vi "Dynamic Channel Lookups.vi"(8 "error in (no error)":errorcluster, 11 "Child Refs":T1[](array[typedef]) format="%.0x") -> (0 "error out":errorcluster, 3 "SLSC Dynamic Inputs":T2[](array[typedef]))   [LabVIEW 2015, in "SLSC-12201 DIO System Explorer.lvlib"]
uses:
  SLSC-12201 DIO System Explorer.lvlib
  Shared/SLSC Dynamic Channel.ctl
  Shared/SLSC Dynamic Channel Type.ctl
  <vilib>/NI Veristand/Custom Device API/Custom Device Item Ref.ctl
  Shared/Constants.vi
  <vilib>/NI Veristand/Custom Device API/Get Item Property (String).vi
  <vilib>/regexp/Match Regular Expression.xnode
  <vilib>/NI Veristand/Custom Device API/Custom Device API.lvlib
  Shared/SLSC-12201 DIO Shared.lvlib
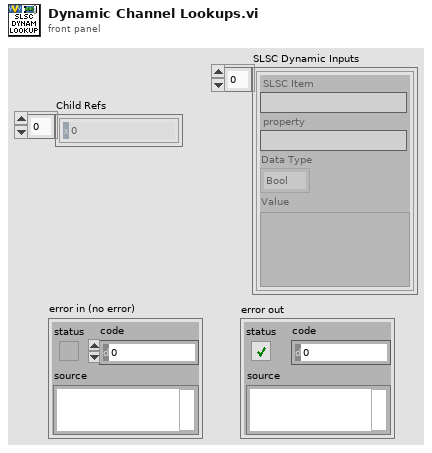
[diagram p1: front panel]
types:
  T1 = typedef "Custom Device API.lvlib/Custom Device Item Ref.ctl" = u64
  T2 = typedef "SLSC-12201 DIO Shared.lvlib/SLSC Dynamic Channel.ctl" = cluster{"SLSC Item":string, "property":string, "Data Type":T3, "Value":variant}
  T3 = typedef "SLSC-12201 DIO Shared.lvlib/SLSC Dynamic Channel Type.ctl" = enum16{"Bool", "Double", "I32", "I64", "String", "U32", "U64", "EnumI32"}
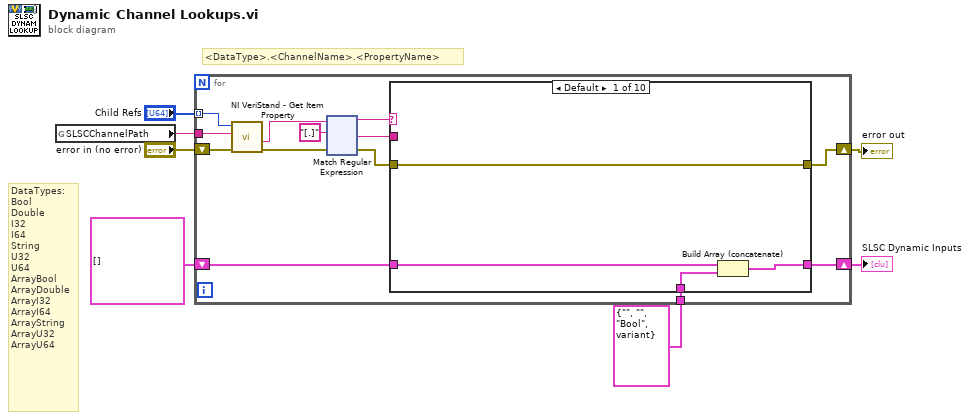
[diagram p0: block diagram]
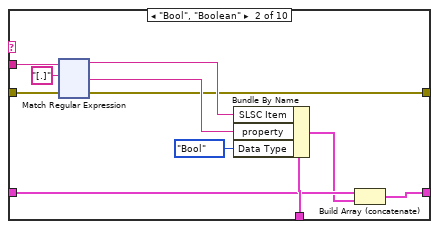
[diagram p2: hidden frame]
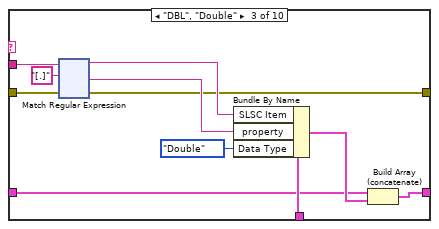
[diagram p3: hidden frame]
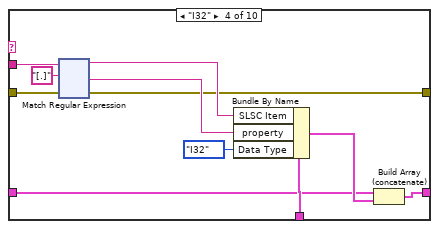
[diagram p4: hidden frame]
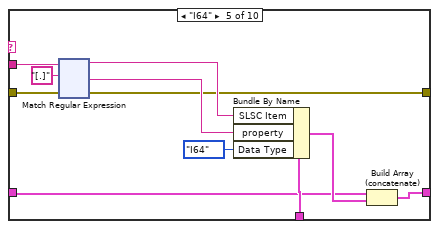
[diagram p5: hidden frame]
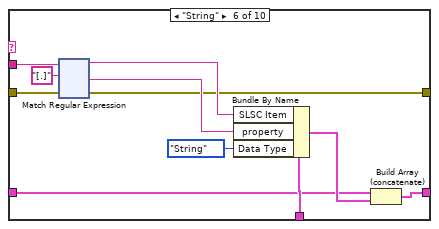
[diagram p6: hidden frame]
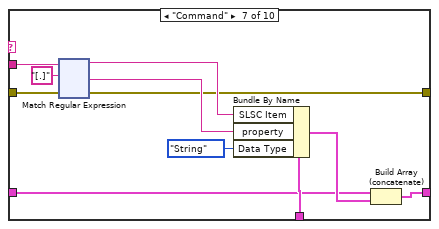
[diagram p7: hidden frame]
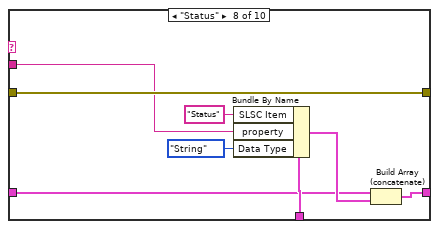
[diagram p8: hidden frame]
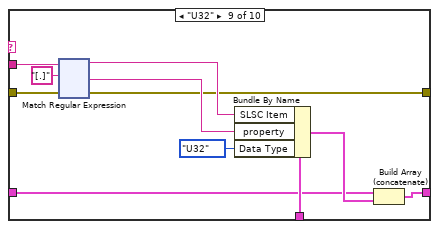
[diagram p9: hidden frame]
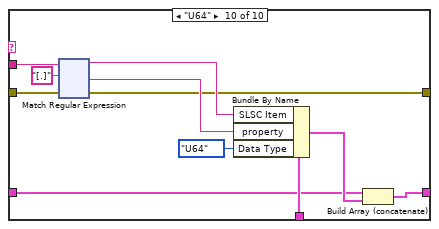
[diagram p10: hidden frame]
diagram:
  # "<DataType>.<ChannelName>.<PropertyName>"
  # "DataTypes:\nBool\nDouble\nI32\nI64\nString\nU32\nU64\nArrayBool\nArrayDouble\nArrayI32\nArrayI64\nArrayString\nArrayU32\nArrayU64"
  n1 = global read "Constants.vi" "SLSCChannelPath"() -> (w6:string)
  n2 = for {
    tunnel: "Child Refs" -> [w20] mode=indexing
    tunnel: w6 -> [w19]
    shift-right: [w8] -> w1
    shift-left: "error in (no error)" -> [w14]
    tunnel: T2 {"SLSC Item"="", "property"="", "Data Type"=enum."Bool", "Value"=variant} ("SLSC Dynamic Channel") -> [w11]
    shift-right: [w9] -> w2
    shift-left: T2[] [] ("SLSC Dynamic Inputs") -> [w10]
    n3 = call-poly <vilib>:"NI VeriStand - Get Item Property.vi"("error in (no error)"=w14, "Property Name"=w19, "Item Ref in"=w20) -> ("error out"=w12:errorcluster, "Value"=w13:string)  [unwired: 5 in, 2 out]
    n4 = xnode "Match Regular Expression"("input string"=w13, "regular expression"="[.]", "error in"=w12) -> ("before match"=w16:string, "after match"=w17:string, "error out"=w18:errorcluster)  [unwired: 3 in, 2 out]
    n5 = case shown="Default" w16 {
      tunnel: w17 -> [_ w34 w159 w284 w409 w534 w659 w776 w792 w917]
      tunnel: w18 -> [w24 w33 w158 w283 w408 w533 w658 w777 w791 w916]
      tunnel: w11 -> [w21 w30 w153 w280 w405 w530 w655 w782 w788 w913]
      tunnel: w10 -> [w23 w29 w151 w277 w401 w527 w652 w779 w784 w909]
      tunnel: [w22 w28 w154 w276 w402 w526 w651 w778 w786 w910] -> w9
      tunnel: [w24 w26 w150 w275 w400 w525 w650 w777 w783 w908] -> w8
      frame Default {
        n6 = Build Array (concatenate)(w23, w21) -> (w22:T2[])
      }
      frame "Bool", "Boolean" {
        n7 = xnode "Match Regular Expression"("input string"=w34, "regular expression"="[.]", "error in"=w33) -> ("before match"=w32:string, "after match"=w31:string, "error out"=w26:errorcluster)  [unwired: 3 in, 2 out]
        n8 = Bundle By Name(cluster=w30, "SLSC Item"=w32, "property"=w31, "Data Type"=SLSC_Dynamic_Channel_Type."Bool") -> (w27:T2)
        n9 = Build Array (concatenate)(w29, w27) -> (w28:T2[])
      }
      frame "DBL", "Double" {
        n10 = xnode "Match Regular Expression"("input string"=w159, "regular expression"="[.]", "error in"=w158) -> ("before match"=w157:string, "after match"=w156:string, "error out"=w150:errorcluster)  [unwired: 3 in, 2 out]
        n11 = Bundle By Name(cluster=w153, "SLSC Item"=w157, "property"=w156, "Data Type"=SLSC_Dynamic_Channel_Type."Double") -> (w152:T2)
        n12 = Build Array (concatenate)(w151, w152) -> (w154:T2[])
      }
      frame "I32" {
        n13 = xnode "Match Regular Expression"("input string"=w284, "regular expression"="[.]", "error in"=w283) -> ("before match"=w282:string, "after match"=w281:string, "error out"=w275:errorcluster)  [unwired: 3 in, 2 out]
        n14 = Bundle By Name(cluster=w280, "SLSC Item"=w282, "property"=w281, "Data Type"=SLSC_Dynamic_Channel_Type."I32") -> (w278:T2)
        n15 = Build Array (concatenate)(w277, w278) -> (w276:T2[])
      }
      frame "I64" {
        n16 = xnode "Match Regular Expression"("input string"=w409, "regular expression"="[.]", "error in"=w408) -> ("before match"=w407:string, "after match"=w406:string, "error out"=w400:errorcluster)  [unwired: 3 in, 2 out]
        n17 = Bundle By Name(cluster=w405, "SLSC Item"=w407, "property"=w406, "Data Type"=SLSC_Dynamic_Channel_Type."I64") -> (w403:T2)
        n18 = Build Array (concatenate)(w401, w403) -> (w402:T2[])
      }
      frame "String" {
        n19 = xnode "Match Regular Expression"("input string"=w534, "regular expression"="[.]", "error in"=w533) -> ("before match"=w532:string, "after match"=w531:string, "error out"=w525:errorcluster)  [unwired: 3 in, 2 out]
        n20 = Bundle By Name(cluster=w530, "SLSC Item"=w532, "property"=w531, "Data Type"=SLSC_Dynamic_Channel_Type."String") -> (w528:T2)
        n21 = Build Array (concatenate)(w527, w528) -> (w526:T2[])
      }
      frame "Command" {
        n22 = xnode "Match Regular Expression"("input string"=w659, "regular expression"="[.]", "error in"=w658) -> ("before match"=w657:string, "after match"=w656:string, "error out"=w650:errorcluster)  [unwired: 3 in, 2 out]
        n23 = Bundle By Name(cluster=w655, "SLSC Item"=w657, "property"=w656, "Data Type"=SLSC_Dynamic_Channel_Type."String") -> (w653:T2)
        n24 = Build Array (concatenate)(w652, w653) -> (w651:T2[])
      }
      frame "Status" {
        n25 = Bundle By Name(cluster=w782, "SLSC Item"="Status", "property"=w776, "Data Type"=SLSC_Dynamic_Channel_Type."String") -> (w780:T2)
        n26 = Build Array (concatenate)(w779, w780) -> (w778:T2[])
      }
      frame "U32" {
        n27 = xnode "Match Regular Expression"("input string"=w792, "regular expression"="[.]", "error in"=w791) -> ("before match"=w790:string, "after match"=w789:string, "error out"=w783:errorcluster)  [unwired: 3 in, 2 out]
        n28 = Bundle By Name(cluster=w788, "SLSC Item"=w790, "property"=w789, "Data Type"=SLSC_Dynamic_Channel_Type."U32") -> (w785:T2)
        n29 = Build Array (concatenate)(w784, w785) -> (w786:T2[])
      }
      frame "U64" {
        n30 = xnode "Match Regular Expression"("input string"=w917, "regular expression"="[.]", "error in"=w916) -> ("before match"=w915:string, "after match"=w914:string, "error out"=w908:errorcluster)  [unwired: 3 in, 2 out]
        n31 = Bundle By Name(cluster=w913, "SLSC Item"=w915, "property"=w914, "Data Type"=SLSC_Dynamic_Channel_Type."U64") -> (w911:T2)
        n32 = Build Array (concatenate)(w909, w911) -> (w910:T2[])
      }
    }
  }
  "SLSC Dynamic Inputs" <- w2
  "error out" <- w1
